vi "GetSystemChannelPaths.vi"(8 "error in (no error)":errorcluster, 10 "System Channel Names in":string[](array[string]), 11 "Workspace Manager Reference in":T1) -> (0 "error out":errorcluster, 1 "System Channel Full Paths out":string[](array[string]), 2 "System Channel Names out":string[](array[string]), 3 "Workspace Manager Reference out":T1)   [LabVIEW 2027, in "VeriStandTestCase.lvclass"]
uses:
  VeriStandTestCase.lvclass
  <vilib>/NI VeriStand/Execution/Workspace/WorkspaceAPI.ctl
  C:/NetCoreDLL/NationalInstruments.VeriStand.ClientAPI.dll
  NetCoreDLL/NationalInstruments.VeriStand.ClientAPI.dll
  <vilib>/NI VeriStand/Execution/Workspace/NI_VS Workspace ExecutionAPI.lvlib
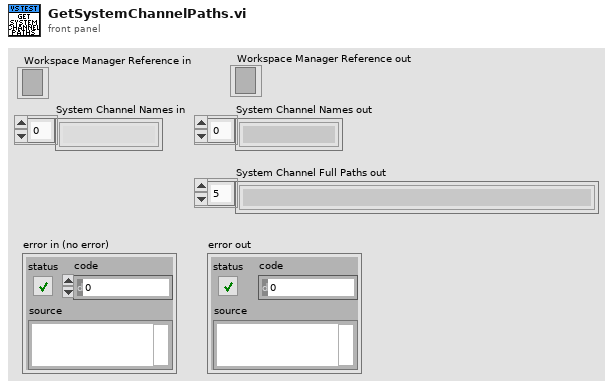
[diagram p1: front panel]
types:
  T1 = typedef "NI_VS Workspace ExecutionAPI.lvlib/WorkspaceAPI.ctl" = refnum<k39>
  T2 = typedef "NI_VS Workspace ExecutionAPI.lvlib/NodeInfo.ctl" = cluster{"Name":string, "FullPath":string, "Type":string, "IsChannel":bool, "Channel":cluster{"Unit":string, "Readable":bool, "Writable":bool, "Faultable":bool, "Scalable":bool, "RowDim":u32, "ColumnDim":u32, "Value Table Names":string[], "Value Table Values":dbl[]}, "IsWaveform":bool, "Waveform":cluster{"DataType":T3}}
  T3 = typedef "NI_VS Workspace ExecutionAPI.lvlib/Waveform Data Type.ctl" = enum16{"Double", "ComplexDouble"}
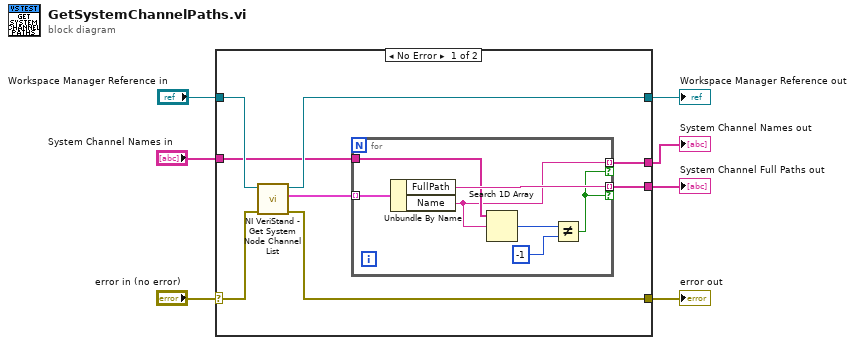
[diagram p0: block diagram]
diagram:
  n1 = case shown="No Error" "error in (no error)" {
    selector: "error in (no error)" -> [w15 w24]
    tunnel: [w11 w24] -> w6
    tunnel: "Workspace Manager Reference in" -> [w14 w23]
    tunnel: [w13 w23] -> w4
    tunnel: [w10 _] -> w3
    tunnel: "System Channel Names in" -> [w9 _]
    tunnel: [w8 _] -> w1
    frame No Error {
      n2 = call <vilib>:"NI VeriStand - Get System Node Channel List.vi"("error in (no error)"=w15, "WorkspaceManager in"=w14) -> ("error out"=w11:errorcluster, "Channels"=w12:T2[], "WorkspaceManager out"=w13:T1)  [unwired: 7 in]
      n3 = for {
        tunnel: w12 -> [w22] mode=indexing
        tunnel: [w21] -> w10 mode=indexing if=w16
        tunnel: w9 -> [w18]
        tunnel: [w17] -> w8 mode=indexing if=w16
        n4 = Unbundle By Name(w22) -> ("FullPath"=w21:string, "Name"=w17:string)
        n5 = Search 1D Array(1D array=w18, element=w17) -> (index of element=w20:i32)  [unwired: 1 in]
        n6 = Not Equal?(x=w20, y=-1) -> (x != y?=w16:bool)
      }
    }
    frame Error {
    }
  }
  "System Channel Full Paths out" <- w3
  "error out" <- w6
  "Workspace Manager Reference out" <- w4
  "System Channel Names out" <- w1
